vi "f44.vi"() -> ()   [LabVIEW 2014]
panel:
  in  "f44":dbl
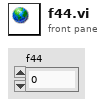
[diagram p1: front panel]
diagram:
